vi "simple db query1.vi"(11 "sql query":string="select distinct count(cycle) from cycleresults where sampletype='s' ;") -> (3 "recordset data":variant[][](array[variant]))   [LabVIEW 2016]
uses:
  <vilib>/addons/database/Connection.llb/DB Tools Open Connec (String).vi
  <vilib>/addons/database/Connection.llb/Conn Execute.vi
  <vilib>/addons/database/Recordset.llb/Rec Fetch Recordset Data (R).vi
  <vilib>/addons/database/Recordset.llb/Rec Destroy - Connection.vi
  <vilib>/addons/database/NI_Database_API.lvlib
panel:
  out "error out 2":errorcluster
  out "data":i32
  out "element":variant
  out "error out":errorcluster
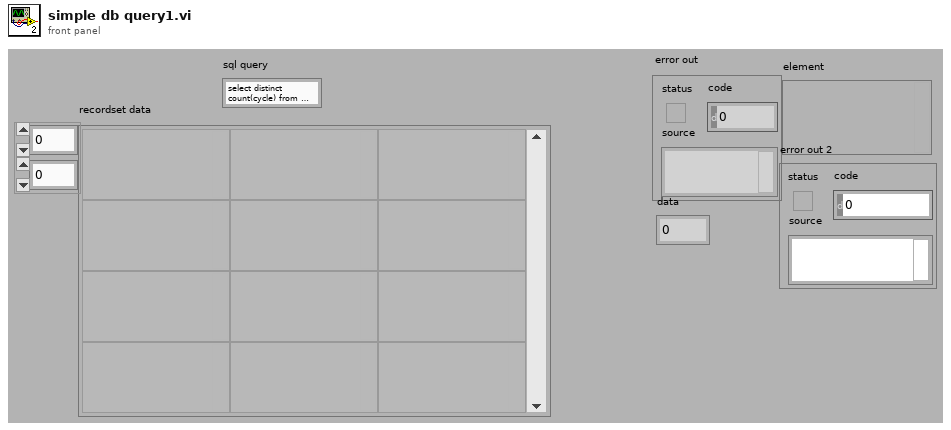
[diagram p1: front panel]
types:
  T1 = typedef "NI_Database_API.lvlib/Conn ObjectReference.ctl" = refnum<k1>
  T2 = typedef "NI_Database_API.lvlib/Rec ObjectReference.ctl" = refnum<k1>
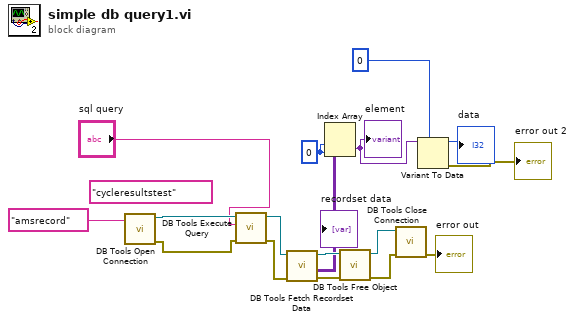
[diagram p0: block diagram]
diagram:
  w5 = 0 ("disabled index (col)")
  (unwired) "cycleresultstest" ("String")
  n1 = call-poly <vilib>:"DB Tools Open Connection.vi"("connection information"="amsrecord") -> ("error out"=w15:errorcluster, "connection reference"=w16:T1)  [unwired: 7 in]
  n2 = call-poly <vilib>:"DB Tools Execute Query.vi"("error in (no error)"=w15, "SQL query"="sql query", "connection reference"=w16) -> ("error out"=w13:errorcluster, "recordset reference"=w14:T2)  [unwired: 5 in]
  n3 = call-poly <vilib>:"DB Tools Fetch Recordset Data.vi"("error in (no error)"=w13, "recordset reference"=w14) -> ("error out"=w12:errorcluster, "recordset data"=w6:variant[][], "recordset reference out"=w11:T2)  [unwired: 3 in]
  "recordset data" <- w6
  n4 = Index Array(array=w6, index (row)=w5, index (col)=w5) -> (element=w4:variant)
  "element" <- w4
  n5 = call-poly <vilib>:"DB Tools Free Object.vi"("error in (no error)"=w12, "recordset reference"=w11) -> ("error out"=w9:errorcluster, "connection reference"=w10:T1)  [unwired: 8 in]
  n6 = call <vilib>:"DB Tools Close Connection.vi"("error in (no error)"=w9, "connection reference"=w10) -> ("error out"=→"error out":errorcluster)  [unwired: 5 in]
  n7 = Variant To Data(type=0 ("disabled index (col)"), Variant=w4) -> (data=→"data":i32, error out=→"error out 2":errorcluster)  [unwired: 1 in]
